vi "Sub Initialize.vi"(8 "error in (no error)":errorcluster, 11 "DAQmx Recorder in":refnum<class "DAQmx Recorder.lvclass">) -> (0 "error out":errorcluster, 2 "Initialize Result":refnum<class "Acquired Result.lvclass">, 3 "DAQmx Recorder out":refnum<class "DAQmx Recorder.lvclass">)   [LabVIEW 2015, in "DAQmx Recorder.lvclass"]
uses:
  DAQmx Recorder.lvclass
  Measure_core/Results/Acquired Result/Acquired Result.lvclass
  DAQmx Recorder.lvclass/DAQmx Recorder.ctl
  NHMFL_Core/Libraries/NI-DAQ/DAQmx Digitizer/DAQmx Digitizer.lvclass/DAQmx Digitizer.ctl
  Read DAQmx Digitizer.lvclass.vi
  NHMFL_Core/Libraries/NI-DAQ/DAQmx Digitizer/Write Configuration.vi
  Write DAQmx Digitizer.lvclass.vi
  Read DAQmx Configuration.vi
  NHMFL_Core/Libraries/NI-DAQ/DAQmx Digitizer/DAQmx Digitizer.lvclass
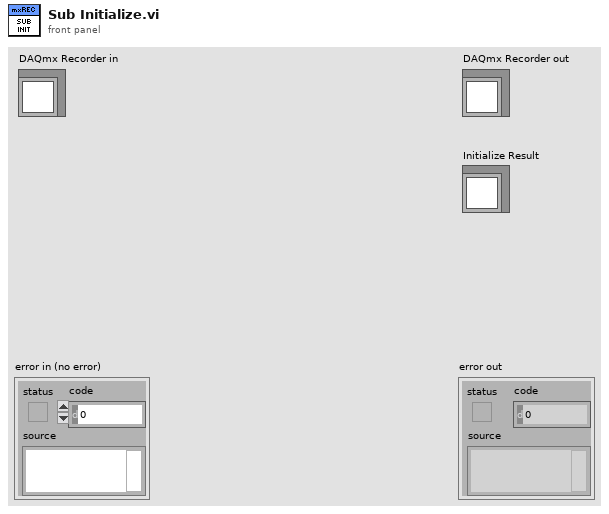
[diagram p1: front panel]
types:
  T1 = typedef "DAQmx Digitizer Configuration.ctl" = cluster{"Pre-trigger duration":dbl, "Post-trigger duration":dbl, "Rate":dbl, "Range":dbl, "Physical Channels":tag, "input configuration":i32, "Channel names":string[]}
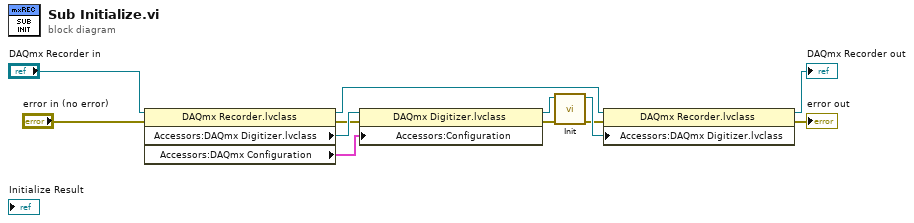
[diagram p0: block diagram]
diagram:
  n1 = property class="DAQmx Recorder.lvclass"(reference="DAQmx Recorder in", error in="error in (no error)") -> (reference out=w5:refnum<class "DAQmx Recorder.lvclass">, error out=w8:errorcluster, "Accessors:DAQmx Digitizer.lvclass"=w11:refnum<class "DAQmx Digitizer.lvclass">, "Accessors:DAQmx Configuration"=w9:T1)
  n2 = property class="DAQmx Digitizer.lvclass"(reference=w11, error in=w8, "Accessors:Configuration"=w9) -> (reference out=w10:refnum<class "DAQmx Digitizer.lvclass">, error out=w7:errorcluster)
  n3 = call-dynamic "Init.vi"("error in (no error)"=w7, "DAQmx Digitizer in"=w10) -> ("error out"=w4:errorcluster, "DAQmx Digitizer out"=w6:refnum<class "DAQmx Digitizer.lvclass">)  [unwired: 8 in]
  n4 = property class="DAQmx Recorder.lvclass"(reference=w5, error in=w4, "Accessors:DAQmx Digitizer.lvclass"=w6) -> (reference out=→"DAQmx Recorder out":refnum<class "DAQmx Recorder.lvclass">, error out=→"error out":errorcluster)
